vi "Get Feature List.vi"(8 "error in":errorcluster) -> (0 "error out":errorcluster, 3 "Feature List":cluster{"name":string, "location":T1}[](array[cluster]))   [LabVIEW 2019, in "route_guide_server.lvlib" / "RouteGuide.lvclass"]
uses:
  RouteGuide.lvclass
  RPC Messages/routeguide_Point.ctl
  route_guide_server.lvlib
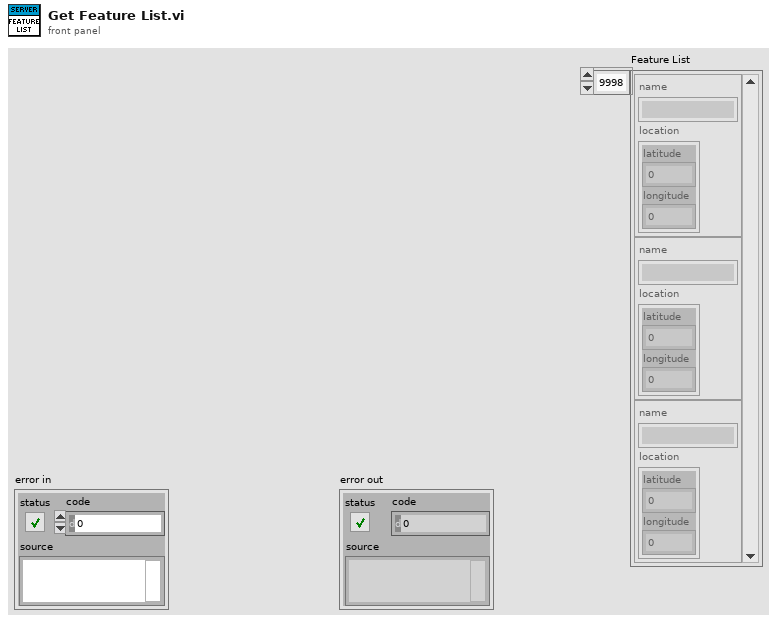
[diagram p1: front panel]
types:
  T1 = typedef "route_guide_server.lvlib/routeguide_Point.ctl" = cluster{"latitude":i32, "longitude":i32}
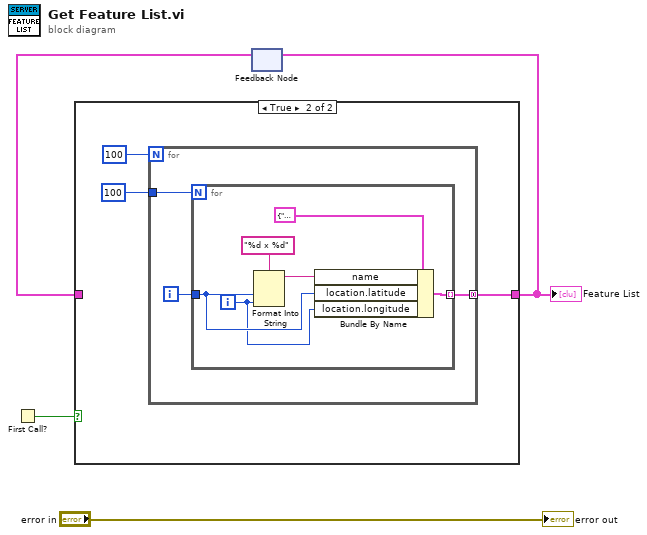
[diagram p0: block diagram]
diagram:
  n1 = First Call?() -> (First Call?: T/F=w3:bool)
  n2 = feedback #1() -> (w1:cluster{"name":string, "location":T1}[])  [unwired: 1 in]
  n3 = case shown="True" w3 {
    tunnel: [w5 w7] -> w2
    tunnel: w1 -> [w5 _]
    frame False {
    }
    frame True {
      n4 = for {
        N: 100 -> [_]
        tunnel: [w10] -> w7 mode=concatenating
        tunnel: 100 -> [w9]
        i -> [w11]
        n5 = for {
          N: w9 -> [_]
          tunnel: w11 -> [w14]
          tunnel: [w12] -> w10 mode=indexing
          i -> [w13]
          n6 = Format Into String(format string="%d x %d", w14, w13) -> (resulting string=w15:string)  [unwired: 2 in, 1 out]
          n7 = Bundle By Name(cluster=cluster{"name":string, "location":T1} {"name"="", "location"={"latitude"=0, "longitude"=0}} ("routeguide_Feature"), "name"=w15, "location.latitude"=w14, "location.longitude"=w13) -> (w12:cluster{"name":string, "location":T1})
        }
      }
    }
  }
  "Feature List" <- w2
  n8 = feedback-in #1(w2) -> ()
  "error out" <- "error in"
